vi "Set Up Terminal for Input Param.vi"(6 "ConPane Terminal Index":u32, 7 "CallLibrary Terminal Index":i32, 8 "Error In":errorcluster, 9 "CalllLibrary Ref":refnum<vi>, 10 "VI Ref":refnum<vi>, 11 "Simple Struct Writer in":refnum<class "Simple Struct Writer.lvclass">) -> (0 "Error Out":errorcluster, 3 "Simple Struct Writer out":refnum<class "Simple Struct Writer.lvclass">)   [LabVIEW 2013, in "Simple Struct Writer.lvclass"]
uses:
  Simple Struct Writer.lvclass
  Simple Struct Writer.lvclass/Simple Struct Writer.ctl
  Abstract Param Writer/Abstract Param Writer.lvclass
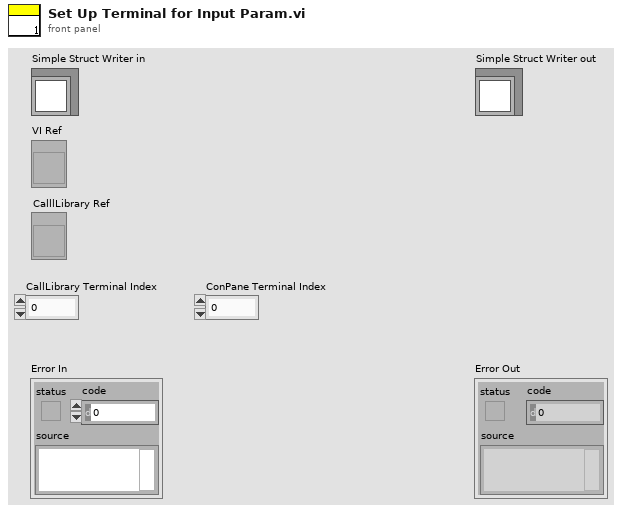
[diagram p1: front panel]
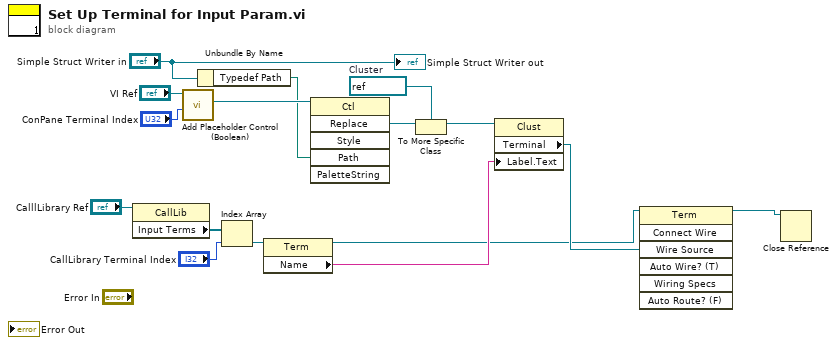
[diagram p0: block diagram]
diagram:
  w5 = refnum<vi> refnum  # Cluster
  n1 = property class="CallLib"(reference="CalllLibrary Ref") -> ("Input Terms"=w15:refnum<vi>[])  [unwired: 1 in, 2 out]
  n2 = call "Add Placeholder Control (Boolean).vi"("ConPane Terminal Index"="ConPane Terminal Index", "VI Ref"="VI Ref") -> ("Control Ref"=w10:refnum<vi>)  [unwired: 9 in]
  n3 = Unbundle By Name("Simple Struct Writer in") -> ("Typedef Path"=w8:path)
  n4 = Index Array(array=w15, index="CallLibrary Terminal Index") -> (element=w13:refnum<vi>)
  n5 = property class="Term"(reference=w13) -> (reference out=w2:refnum<vi>, "Name"=w4:string)  [unwired: 1 in, 1 out]
  n6 = invoke class="Ctl" method="Replace"(reference=w10, "Path"=w8) -> ("Replace"=w7:refnum<vi>)  [unwired: 4 in, 5 out]
  n7 = To More Specific Class(target class=w5, reference=w7) -> (specific class reference=w6:refnum<vi>)  [unwired: 1 in, 1 out]
  n8 = property class="Clust"(reference=w6, "Label.Text"=w4) -> ("Terminal"=w3:refnum<vi>)  [unwired: 1 in, 2 out]
  n9 = invoke class="Term" method="Connect Wire"(reference=w2, "Wire Source"=w3) -> (reference out=w1:refnum<vi>)  [unwired: 5 in, 6 out]
  n10 = Close Reference(reference=w1) -> ()  [unwired: 1 in, 1 out]
  "Simple Struct Writer out" <- "Simple Struct Writer in"
